vi "SECoP-nodeComplete.vi"(8 "error in (no error)":errorcluster, 11 "DLL path (in)":T1) -> (0 "error out":errorcluster, 3 "DLL path (out)":T1)   [LabVIEW 2023, in "SECoP.lvlib"]
doc: "Call <b>\"SECoP-nodeComplete.vi\"</b> to inform the SEC node that it is complete. This function makes some checks and on success, it opens the TCP port and marks the node that you cannot change its structure. The SEC node is not usable before this call does not return an error.\n\n<b>DLL path</b> input and output of cluster from \"SECoP-Initialize.vi\""
uses:
  SECoP.lvlib
  SECoP-libraries.ctl
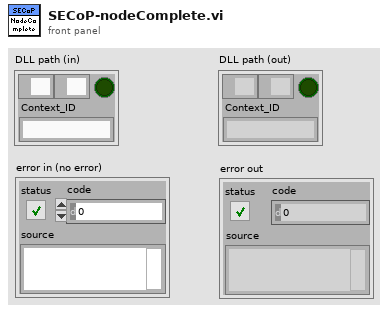
[diagram p1: front panel]
types:
  T1 = typedef "SECoP.lvlib/SECoP-libraries.ctl" = cluster{"serverDLL":path, "variantDLL":path, "cleanup_mode":bool, "Context_ID":string}
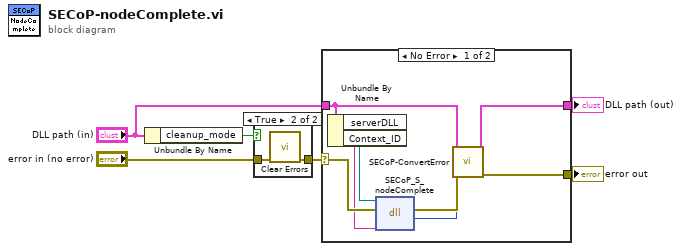
[diagram p0: block diagram]
diagram:
  n1 = Unbundle By Name("DLL path (in)") -> ("cleanup_mode"=w3:bool)
  n2 = case shown="True" w3 {
    tunnel: "error in (no error)" -> [w7 w9]
    tunnel: [w7 w8] -> w1
    frame False {
    }
    frame True {
      n3 = call <vilib>:"Clear Errors.vi"("error in (no error)"=w9) -> ("error out"=w8:errorcluster)  [unwired: 5 in, 1 out]
    }
  }
  n4 = case shown="No Error" w1 {
    selector: w1 -> [w15 w18]
    tunnel: "DLL path (in)" -> [w12 w19]
    tunnel: [w16 w19] -> w5
    tunnel: [w17 w18] -> w4
    frame No Error {
      n5 = Unbundle By Name(w12) -> ("serverDLL"=w11:path, "Context_ID"=w10:string)
      n6 = dll-call lib="C:/Users/user/Desktop/x86_64/SECoP64.dll" fn="SECoP_S_nodeComplete"(path in=w11, error in=w15, "szContextID"=w10) -> (error out=w14:errorcluster, "return type"=w13:i32)  [unwired: 2 in, 1 out]
      n7 = call "SECoP-ConvertError.vi"("return code"=w13, "error in (no error)"=w14, "DLL path (in)"=w12) -> ("error out"=w17:errorcluster, "DLL path (out)"=w16:T1)  [unwired: 7 in]
    }
    frame Error {
    }
  }
  "DLL path (out)" <- w5
  "error out" <- w4
